vi "Get Wheel Motors Velocity.vi"(8 "error in (no error)":errorcluster, 11 "KUKA youBot platform in":refnum<class "NI_Robotics_KUKA youBot Platform.lvclass">) -> (0 "error out":errorcluster, 2 "ccw velocity (rad/s)":dbl[](array[numeric]), 3 "KUKA youBot platform out":refnum<class "NI_Robotics_KUKA youBot Platform.lvclass">)   [LabVIEW 2017, in "NI_Robotics_KUKA youBot Host.lvlib" / "NI_Robotics_KUKA youBot Platform.lvclass"]
doc: "Gets the sensed motors velocity of the wheels of a KUKA youBot mobile platform."
uses:
  <vilib>/robotics/KUKA youBot/Basic Device/Mobile Platform/NI_Robotics_KUKA youBot Platform.lvclass
  <vilib>/robotics/KUKA youBot/Basic Device/Mobile Platform/NI_Robotics_KUKA youBot Platform.lvclass/NI_Robotics_KUKA youBot Platform.ctl
  <vilib>/robotics/KUKA youBot/Motor/Wheel Motor/NI_Robotics_KUKA youBot Wheel Motor.lvclass
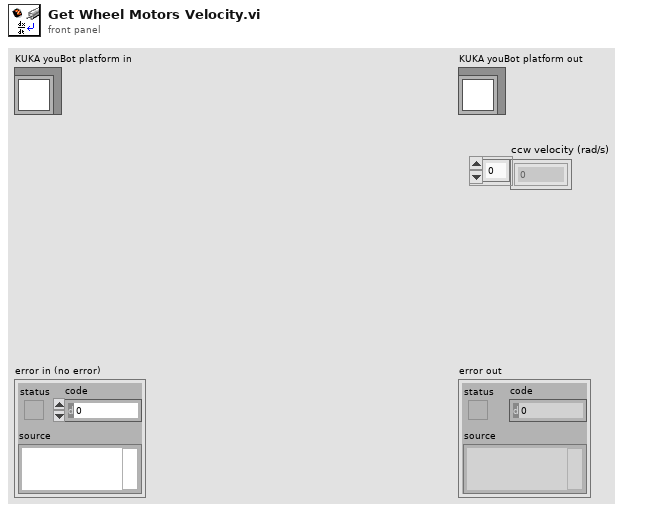
[diagram p1: front panel]
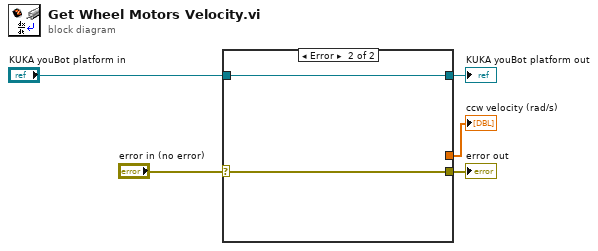
[diagram p0: block diagram]
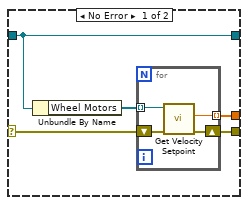
[diagram p2: hidden frame]
diagram:
  n1 = case shown="Error" "error in (no error)" {
    selector: "error in (no error)" -> [w7 w15]
    tunnel: [w6 w15] -> w4
    tunnel: [w10 w16] -> w2
    tunnel: "KUKA youBot platform in" -> [w10 w16]
    tunnel: [w8 _] -> w1
    frame No Error {
      n2 = Unbundle By Name(w10) -> ("Wheel Motors"=w9:refnum<class "NI_Robotics_KUKA youBot Wheel Motor.lvclass">[])
      n3 = for {
        tunnel: w9 -> [w14] mode=indexing
        tunnel: [w13] -> w8 mode=indexing
        shift-right: [w11] -> w6
        shift-left: w7 -> [w12]
        n4 = call-dynamic "Get Velocity Setpoint.vi"("error in (no error)"=w12, "KUKA youBot wheel motor in"=w14) -> ("error out"=w11:errorcluster, "CCW velocity (rad/s)"=w13:dbl)  [unwired: 7 in, 1 out]
      }
    }
    frame Error {
    }
  }
  "error out" <- w4
  "KUKA youBot platform out" <- w2
  "ccw velocity (rad/s)" <- w1
